vi "reCalibratePlatforms.vi"   [LabVIEW 2017]
doc: "The load cells output a voltage even when no weight is present on the platform. This needs to be measured so that it can be subtracted from subsequent measurements of platform load. The VI will output a spreadsheet saved in the current folder."
uses:
  <vilib>/Utility/file.llb/Write Delimited Spreadsheet (string).vi
  <vilib>/Utility/file.llb/Write Delimited Spreadsheet (DBL).vi
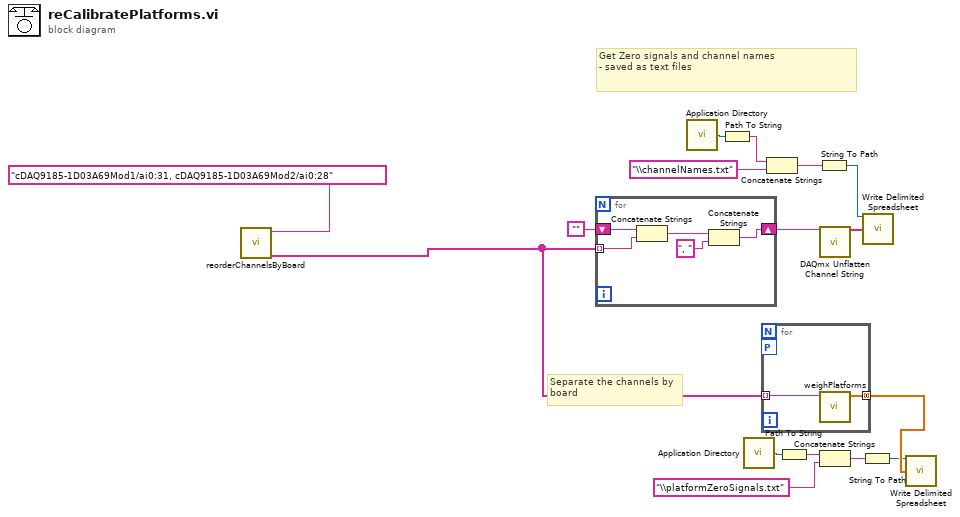
[diagram p0: block diagram]
diagram:
  # "Separate the channels by\nboard"
  # "Get Zero signals and channel names \n- saved as text files"
  n1 = call "reorderChannelsByBoard.vi"("DAQmx \nPhysical Channel"=tag "cDAQ9185-1D03A69Mod1/ai0:31, cDAQ9185-1D03A69Mod2/ai0:28" ("DAQmx \nPhysical Channel")) -> ("Separated inputs\nas strings"=w15:string[])  [unwired: 8 in, 2 out]
  n2 = for {
    shift-right: [w20] -> w12
    shift-left: "" -> [w21]
    tunnel: w15 -> [w17] mode=indexing
    n3 = Concatenate Strings(w21, w17) -> (w19:string)
    n4 = Concatenate Strings(w19, ", ") -> (w20:string)
  }
  n5 = call <vilib>:"Application Directory.vi"() -> ("Application Directory"=w9:path)
  n6 = Path To String(path=w9) -> (string=w8:string)
  n7 = call <vilib>:"Application Directory.vi"() -> ("Application Directory"=w4:path)
  n8 = for {
    workers-P: _ -> [_]
    tunnel: [w22] -> w14 mode=concatenating
    tunnel: w15 -> [w23] mode=indexing
    n9 = call "weighPlatforms.vi"("DAQmx Physical Channel"=w23) -> ("load cell\nsignal"=w22:dbl[])  [unwired: 10 in]
  }
  n10 = Concatenate Strings(w8, "\\channelNames.txt") -> (w7:string)
  n11 = Path To String(path=w4) -> (string=w3:string)
  n12 = String To Path(string=w7) -> (path=w6:path)
  n13 = call <vilib>:"DAQmx Unflatten Channel String.vi"("names in"=w12) -> ("names out"=w11:string[])  [unwired: 13 in, 1 out]
  n14 = Concatenate Strings(w3, "\\platformZeroSignals.txt") -> (w2:string)
  n15 = String To Path(string=w2) -> (path=w1:path)
  n16 = call-poly <vilib>:"Write Delimited Spreadsheet.vi"("file path (dialog if empty)"=w6, "1D data"=w11) -> ()  [unwired: 12 in, 2 out]
  n17 = call-poly <vilib>:"Write Delimited Spreadsheet.vi"("file path (dialog if empty)"=w1, "1D data"=w14) -> ()  [unwired: 12 in, 2 out]
